vi "Measure (Calling Interface).vi"(10 "t":dbl, 11 "Sinusoid in":refnum<class "Sinusoid.lvclass">) -> (2 "y":dbl)   [LabVIEW 2024]
uses:
  Interfaces/Sinusoid/Sinusoid.lvclass
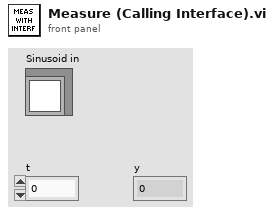
[diagram p1: front panel]
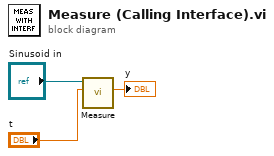
[diagram p0: block diagram]
diagram:
  n1 = call-dynamic "Measure.vi"("t (seconds)"="t", "Sinusoid in"="Sinusoid in") -> ("y"=→"y":dbl)  [unwired: 8 in, 1 out]
